vi "EOL CAN_Disable_Parametric_Mode.vi"(8 "Error in":errorcluster, 10 "Read Session in":refnum<k21>, 11 "Write Session in":refnum<k21>) -> (0 "Error out":errorcluster, 2 "debug log":string[][](array[string]), 3 "Response Good?":bool)   [LabVIEW 2018]
uses:
  <vilib>/xnet/xnet.llb/XNET Frame CAN.ctl
  <vilib>/xnet/xnet.llb/XNET Frame Type CAN.ctl
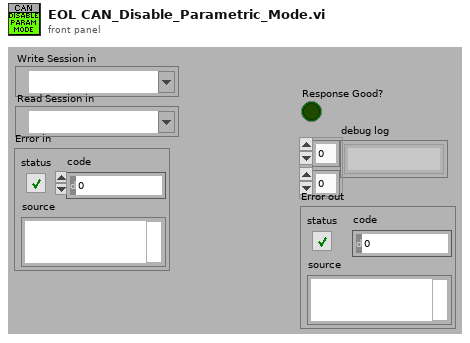
[diagram p1: front panel]
types:
  T1 = typedef "XNET Frame CAN.ctl" = cluster{"timestamp":timestamp, "payload":u8[], "identifier":u32, "type":T2, "extended?":bool, "echo?":bool}
  T2 = typedef "XNET Frame Type CAN.ctl" = u8
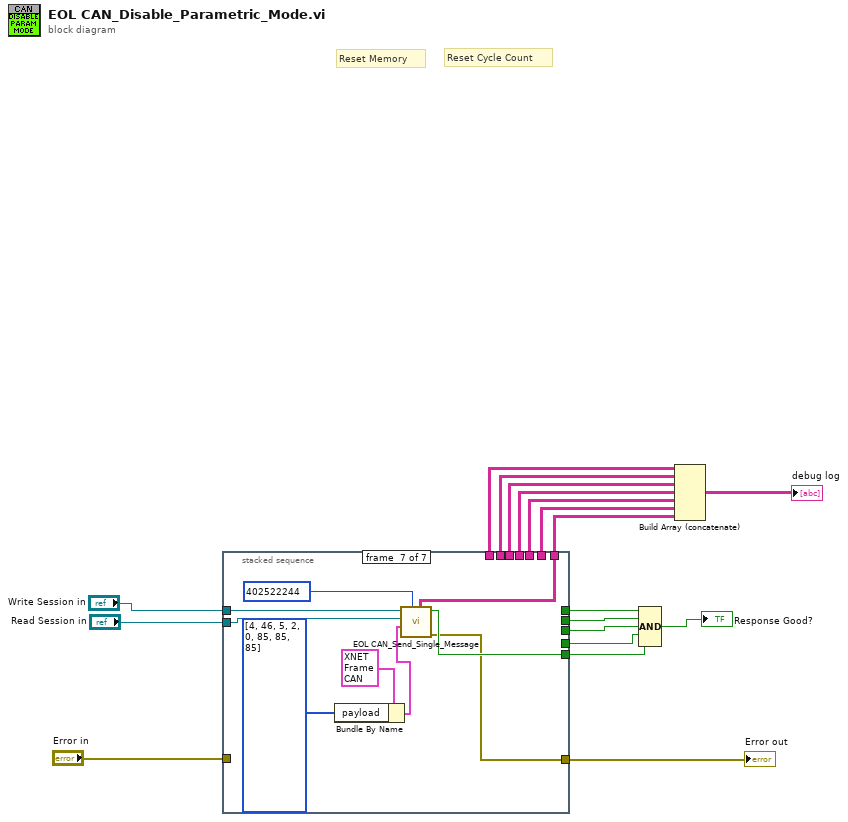
[diagram p0: block diagram]
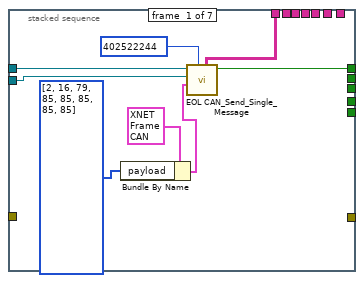
[diagram p2: hidden frame]
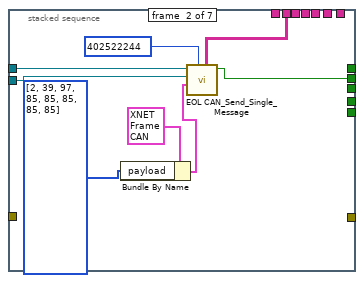
[diagram p3: hidden frame]
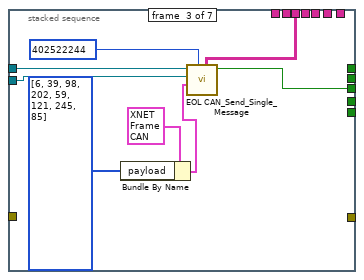
[diagram p4: hidden frame]
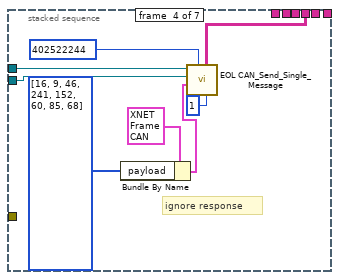
[diagram p5: hidden frame]
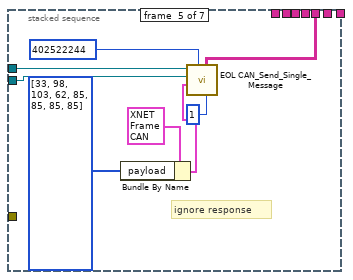
[diagram p6: hidden frame]
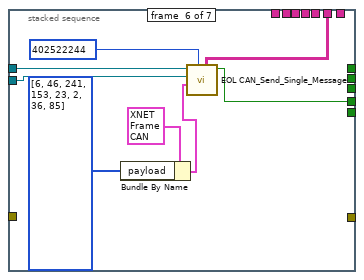
[diagram p7: hidden frame]
diagram:
  # "Reset Memory"
  # "Reset Cycle Count"
  n1 = stacked-sequence {
    tunnel: [w26 _ _ _ _ _ _] -> w18
    tunnel: [w25 _ _ _ _ _ _] -> w16
    tunnel: "Write Session in" -> [w24 w34 w42 w50 w58 w66 w75]
    tunnel: "Read Session in" -> [w23 w33 w41 w49 w57 w65 w74]
    tunnel: [_ w28 _ _ _ _ _] -> w12
    tunnel: [_ w27 _ _ _ _ _] -> w11
    tunnel: [_ _ w36 _ _ _ _] -> w10
    tunnel: [_ _ w35 _ _ _ _] -> w9
    tunnel: [_ _ _ w43 _ _ _] -> w3
    tunnel: [_ _ _ _ _ w60 _] -> w8
    tunnel: [_ _ _ _ _ _ w69] -> w7
    tunnel: [_ _ _ _ _ _ w68] -> w6
    tunnel: "Error in" -> [_ _ _ _ _ _ _]
    tunnel: [_ _ _ _ _ _ w67] -> w4
    tunnel: [_ _ _ _ w51 _ _] -> w2
    tunnel: [_ _ _ _ _ w59 _] -> w1
    frame #0 {
      n2 = Bundle By Name(cluster=T1 {"timestamp"=timestamp(0 s since 1904-01-01), "payload"=[2, 39, 3, 85, 85, 85, 85, 85], "identifier"=402391172, "type"=8, "extended?"=TRUE, "echo?"=FALSE} ("Tx CAN frame"), "payload"=u8[] [2, 16, 79, 85, 85, 85, 85, 85] ("Transmit Data 2")) -> (w21:T1)
      n3 = call "EOL CAN_Send_Single_Message.vi"("Rx Arbitration Id"=u32 402522244, "Tx CAN frame"=w21, "Read Session in"=w23, "Write Session in"=w24) -> ("Response Good?"=w26:bool, "TxRx Data"=w25:string[][])  [unwired: 3 in, 3 out]
    }
    frame #1 {
      n4 = Bundle By Name(cluster=T1 {"timestamp"=timestamp(0 s since 1904-01-01), "payload"=[2, 39, 3, 85, 85, 85, 85, 85], "identifier"=402391172, "type"=8, "extended?"=TRUE, "echo?"=FALSE} ("Tx CAN frame"), "payload"=u8[] [2, 39, 97, 85, 85, 85, 85, 85] ("Transmit Data 2")) -> (w32:T1)
      n5 = call "EOL CAN_Send_Single_Message.vi"("Rx Arbitration Id"=u32 402522244, "Tx CAN frame"=w32, "Read Session in"=w33, "Write Session in"=w34) -> ("Response Good?"=w27:bool, "TxRx Data"=w28:string[][])  [unwired: 3 in, 3 out]
    }
    frame #2 {
      n6 = Bundle By Name(cluster=T1 {"timestamp"=timestamp(0 s since 1904-01-01), "payload"=[2, 39, 3, 85, 85, 85, 85, 85], "identifier"=402391172, "type"=8, "extended?"=TRUE, "echo?"=FALSE} ("Tx CAN frame"), "payload"=u8[] [6, 39, 98, 202, 59, 121, 245, 85] ("Transmit Data 2")) -> (w40:T1)
      n7 = call "EOL CAN_Send_Single_Message.vi"("Rx Arbitration Id"=u32 402522244, "Tx CAN frame"=w40, "Read Session in"=w41, "Write Session in"=w42) -> ("Response Good?"=w35:bool, "TxRx Data"=w36:string[][])  [unwired: 3 in, 3 out]
    }
    frame #3 {
      # "ignore response"
      n8 = Bundle By Name(cluster=T1 {"timestamp"=timestamp(0 s since 1904-01-01), "payload"=[2, 39, 3, 85, 85, 85, 85, 85], "identifier"=402391172, "type"=8, "extended?"=TRUE, "echo?"=FALSE} ("Tx CAN frame"), "payload"=u8[] [16, 9, 46, 241, 152, 60, 85, 68] ("Transmit Data 2")) -> (w48:T1)
      n9 = call "EOL CAN_Send_Single_Message.vi"("Retries"=1, "Rx Arbitration Id"=u32 402522244, "Tx CAN frame"=w48, "Read Session in"=w49, "Write Session in"=w50) -> ("TxRx Data"=w43:string[][])  [unwired: 2 in, 4 out]
    }
    frame #4 {
      # "ignore response"
      n10 = Bundle By Name(cluster=T1 {"timestamp"=timestamp(0 s since 1904-01-01), "payload"=[2, 39, 3, 85, 85, 85, 85, 85], "identifier"=402391172, "type"=8, "extended?"=TRUE, "echo?"=FALSE} ("Tx CAN frame"), "payload"=u8[] [33, 98, 103, 62, 85, 85, 85, 85] ("Transmit Data 2")) -> (w56:T1)
      n11 = call "EOL CAN_Send_Single_Message.vi"("Retries"=1, "Rx Arbitration Id"=u32 402522244, "Tx CAN frame"=w56, "Read Session in"=w57, "Write Session in"=w58) -> ("TxRx Data"=w51:string[][])  [unwired: 2 in, 4 out]
    }
    frame #5 {
      n12 = Bundle By Name(cluster=T1 {"timestamp"=timestamp(0 s since 1904-01-01), "payload"=[2, 39, 3, 85, 85, 85, 85, 85], "identifier"=402391172, "type"=8, "extended?"=TRUE, "echo?"=FALSE} ("Tx CAN frame"), "payload"=u8[] [6, 46, 241, 153, 23, 2, 36, 85] ("Transmit Data 2")) -> (w64:T1)
      n13 = call "EOL CAN_Send_Single_Message.vi"("Rx Arbitration Id"=u32 402522244, "Tx CAN frame"=w64, "Read Session in"=w65, "Write Session in"=w66) -> ("Response Good?"=w60:bool, "TxRx Data"=w59:string[][])  [unwired: 3 in, 3 out]
    }
    frame #6 {
      n14 = Bundle By Name(cluster=T1 {"timestamp"=timestamp(0 s since 1904-01-01), "payload"=[2, 39, 3, 85, 85, 85, 85, 85], "identifier"=402391172, "type"=8, "extended?"=TRUE, "echo?"=FALSE} ("Tx CAN frame"), "payload"=u8[] [4, 46, 5, 2, 0, 85, 85, 85] ("Transmit Data 2")) -> (w73:T1)
      n15 = call "EOL CAN_Send_Single_Message.vi"("Rx Arbitration Id"=u32 402522244, "Tx CAN frame"=w73, "Read Session in"=w74, "Write Session in"=w75) -> ("Error out"=w67:errorcluster, "Response Good?"=w68:bool, "TxRx Data"=w69:string[][])  [unwired: 3 in, 2 out]
    }
  }
  "Error out" <- w4
  n16 = Compound Arithmetic op=AND(w18, w11, w9, w8, w6) -> (→"Response Good?":bool)
  n17 = Build Array (concatenate)(w16, w12, w10, w3, w2, w1, w7) -> (→"debug log":string[][])
